vi "Read Force rebuild.vi"(11 "SolutionBuilder in":refnum<class "SolutionBuilder.lvclass">) -> (2 "Force rebuild":bool, 3 "SolutionBuilder out":refnum<class "SolutionBuilder.lvclass">)   [LabVIEW 2019, in "SolutionBuilder.lvlib" / "SolutionBuilder.lvclass"]
uses:
  SolutionBuilder.lvclass
  SolutionBuilder.lvclass/SolutionBuilder.ctl
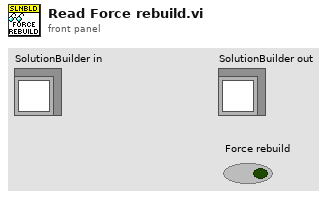
[diagram p1: front panel]
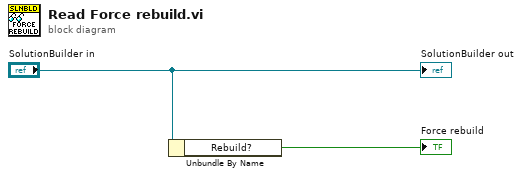
[diagram p0: block diagram]
diagram:
  n1 = Unbundle By Name("SolutionBuilder in") -> ("Rebuild?"=→"Force rebuild":bool)
  "SolutionBuilder out" <- "SolutionBuilder in"
